vi "Configure Channels.vi"(8 "error in (no error)":errorcluster, 11 "object in":refnum<class "Fetch Waveforms CFG.lvclass">) -> (0 "error out":errorcluster, 3 "object out":refnum<class "Fetch Waveforms CFG.lvclass">)   [LabVIEW 2023, in "Scope Simulated CFGs.lvlib" / "Fetch Waveforms CFG.lvclass"]
uses:
  Fetch Waveforms CFG.lvclass
  Fetch Waveforms CFG.lvclass/Fetch Waveforms CFG.ctl
  <vilib>/Utility/error.llb/Error Cluster From Error Code.vi
  <vilib>/ErrorRing/Error Ring.xnode
  7cfe5669-d9a9-4cf8-b296-982c00835eb7.vi
  Configuration JSON Base/CFG JSON Base.lvclass
panel:
  out "Data":T1(array[cluster])
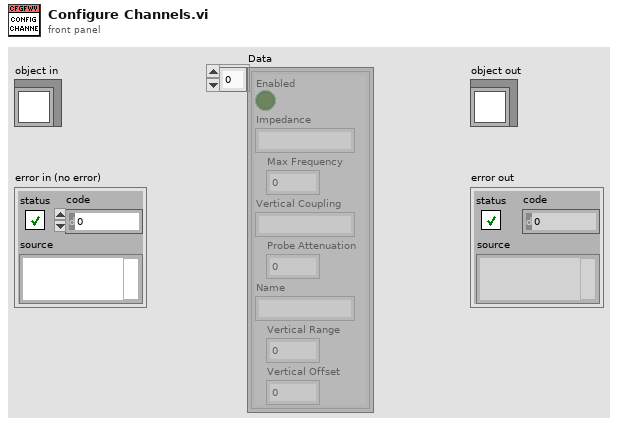
[diagram p1: front panel]
types:
  T1 = cluster{"Enabled":bool, "Impedance":string, "Max Frequency":dbl, "Vertical Coupling":string, "Probe Attenuation":dbl, "Name":string, "Vertical Range":dbl, "Vertical Offset":dbl}[]
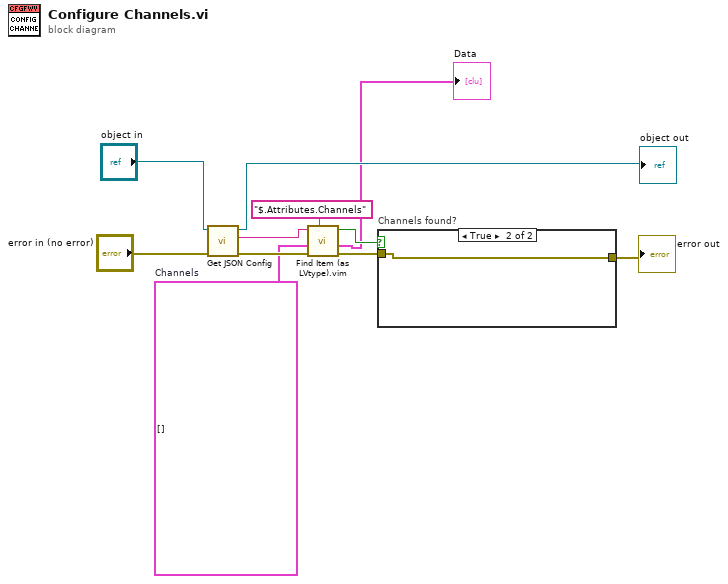
[diagram p0: block diagram]
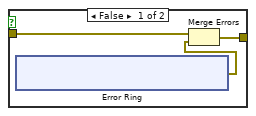
[diagram p2: hidden frame]
diagram:
  w7 = T1 []  # Channels
  n1 = call "Get JSON Config.vi"("error in (no error)"="error in (no error)", "CFG Base in"="object in") -> ("error out"=w8:errorcluster, "<JSON>Config>"=w9:string, "CFG Base out"=→"object out":refnum<class "Fetch Waveforms CFG.lvclass">)  [unwired: 7 in]
  n2 = call "Find Item (as LVtype).vim"("$Path or Item Name"="$.Attributes.Channels", "error in (no error)"=w8, "Data Type and Default Value"=w7, "JSON"=w9) -> ("error out"=w5:errorcluster, "Data"=→"Data":T1, "Found"=w6:bool)  [unwired: 4 in, 1 out]
  n3 = case "Channels found?" shown="True" w6 {
    tunnel: [w14 w20] -> w2
    tunnel: w5 -> [w12 w20]
    frame False {
      n4 = xnode "Error Ring"() -> ("error out"=w13:errorcluster)
      n5 = Merge Errors(w12, w13) -> (w14:errorcluster)
    }
    frame True {
    }
  }
  "error out" <- w2
